vi "StepVoltage.vi"() -> ()   [LabVIEW 2014]
uses:
  <vilib>/Utility/error.llb/DialogType.ctl
  <vilib>/DAQmx/write.llb/DAQmx Write (Analog 1D Wfm NChan NSamp).vi
  <vilib>/DAQmx/create/channels.llb/DAQmx Create Channel (AO-Voltage-Basic).vi
  <vilib>/DAQmx/configure/timing.llb/DAQmx Timing (Sample Clock).vi
  <vilib>/DAQmx/miscellaneous.llb/DAQmx Fill In Error Info.vi
  <resource>/objmgr/daqmx.rc
panel:
  in  "samples per channel":i32=87751
  in  "Sample Rate":dbl=1000.0
  in  "Sample Clock Source":tag="OnboardClock"
  in  "Max Voltage":dbl=10.0
  in  "Min Voltage":dbl=-10.0
  in  "Physical Channel(s)":tag="Dev1/ao0,Dev1/ao1,Dev1/ao3"
  out "Actual Sample Rate":dbl=1000.0 format="%0.2f"
  in  "Stop":bool
  out "Waveform Graph 2":dynamicdata(graph)
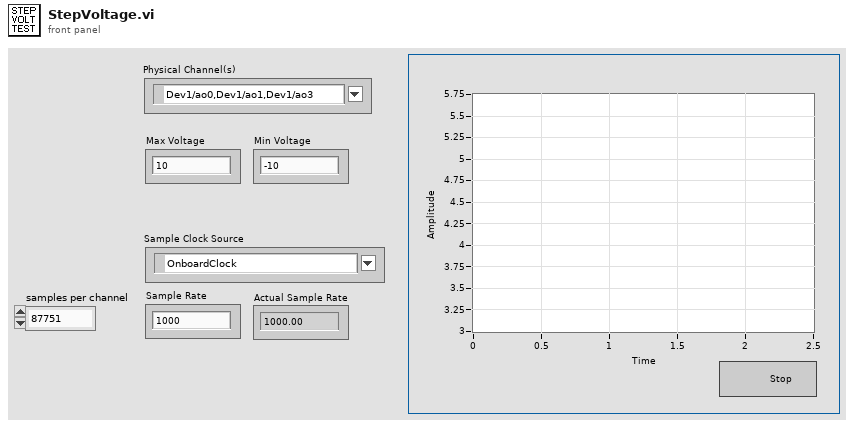
[diagram p1: front panel]
types:
  T1 = typedef "DialogType.ctl" = u16
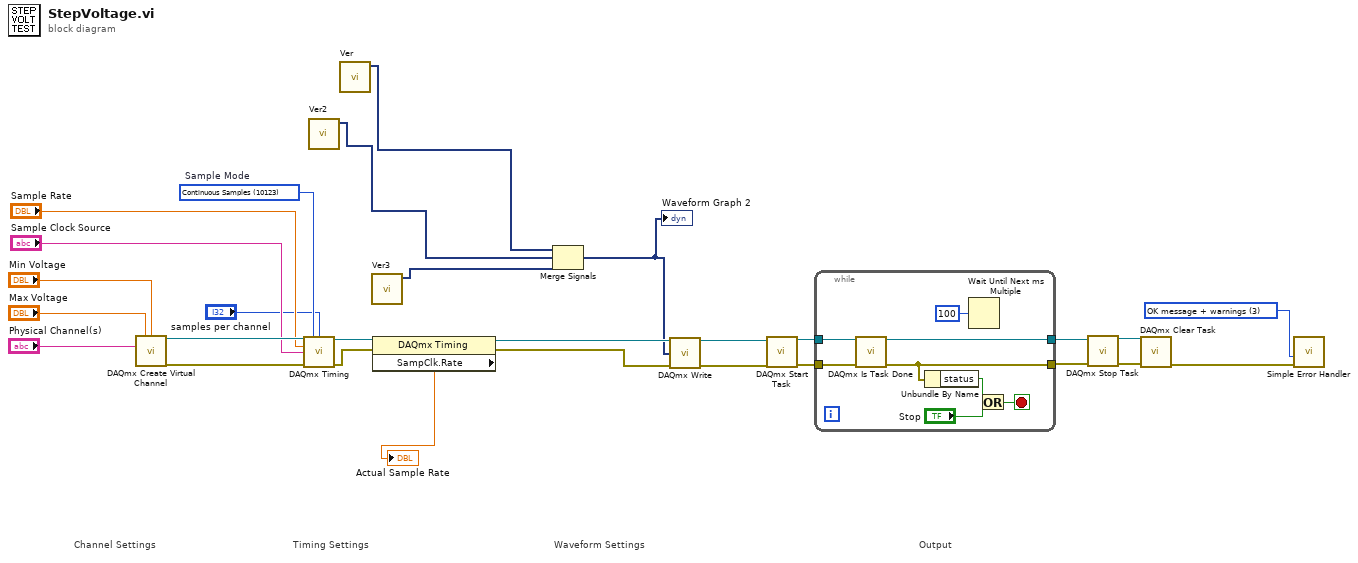
[diagram p0: block diagram]
diagram:
  w8 = T1 3 items=["no dialog", "OK message", "continue or stop message", "OK message + warnings", "continue/stop + warnings"] ("type of dialog (OK msg:1)")
  w26 = 10123 items=["Finite Samples"=10178, "Continuous Samples"=10123, "Hardware Timed Single Point"=12522]  # Sample Mode
  # "Output"
  # "Waveform Settings"
  # "Timing Settings"
  # "Channel Settings"
  n1 = call-poly <vilib>:"DAQmx Create Virtual Channel.vi"("maximum value"="Max Voltage", "minimum value"="Min Voltage", "physical channels"="Physical Channel(s)") -> ("task out"=w24:refnum<k21>, "error out"=w25:errorcluster)  [unwired: 11 in]
  n2 = call-poly <vilib>:"DAQmx Timing.vi"("task/channels in"=w24, "sample mode"=w26, "samples per channel"="samples per channel", "rate"="Sample Rate", "source"="Sample Clock Source", "error in"=w25) -> ("task out"=w28:refnum<k21>, "error out"=w27:errorcluster)  [unwired: 8 in]
  n3 = call "Ver2"() -> ("Signal"=w2:dynamicdata)  [unwired: 9 in, 2 out]
  n4 = call "Ver"() -> ("Signal"=w3:dynamicdata)  [unwired: 9 in, 2 out]
  n5 = call "Ver3"() -> ("Signal"=w1:dynamicdata)  [unwired: 9 in, 2 out]
  n6 = property class="DAQmx Timing"(reference=w28, error in=w27) -> (reference out=w7:refnum<k21>, error out=w6:errorcluster, "SampClk.Rate"=→"Actual Sample Rate":dbl)
  n7 = Merge Signals(w3, w2, w1) -> (w5:dynamicdata)
  "Waveform Graph 2" <- w5
  n8 = call-poly <vilib>:"DAQmx Write.vi"("task/channels in"=w7, "data"=w5, "error in"=w6) -> ("task out"=w14:refnum<k21>, "error out"=w13:errorcluster)  [unwired: 10 in, 1 out]
  n9 = call <vilib>:"DAQmx Start Task.vi"("task/channels in"=w14, "error in"=w13) -> ("task out"=w23:refnum<k21>, "error out"=w22:errorcluster)  [unwired: 12 in]
  n10 = while {
    tunnel: w23 -> [w36]
    tunnel: w22 -> [w35]
    tunnel: [w32] -> w9
    tunnel: [w33] -> w10
    stop <- w34 stop-if-true
    n11 = call <vilib>:"DAQmx Is Task Done.vi"("task/channels in"=w36, "error in"=w35) -> ("task out"=w33:refnum<k21>, "error out"=w32:errorcluster)  [unwired: 11 in, 1 out]
    n12 = Unbundle By Name(w32) -> ("status"=w31:bool)
    n13 = Wait Until Next ms Multiple(millisecond multiple=u32 100) -> ()  [unwired: 1 out]
    n14 = Or(x=w31, y="Stop") -> (x .or. y?=w34:bool)
  }
  n15 = call <vilib>:"DAQmx Stop Task.vi"("task/channels in"=w10, "error in"=w9) -> ("task out"=w12:refnum<k21>, "error out"=w11:errorcluster)  [unwired: 12 in]
  n16 = call <vilib>:"DAQmx Clear Task.vi"("task in"=w12, "error in"=w11) -> ("error out"=w21:errorcluster)  [unwired: 13 in]
  n17 = call <vilib>:"Simple Error Handler.vi"("type of dialog (OK msg:1)"=w8, "error in (no error)"=w21) -> ()  [unwired: 3 in, 5 out]
